vi "BodeFrequencyResponseAnalyzer.vi"() -> ()   [LabVIEW 2026]
doc: "Measures the magnitude and phase response of an electronic filter using synchronized analog generation and acquisition with NI-DAQmx."
uses:
  <vilib>/Utility/error.llb/DialogType.ctl
  <vilib>/DAQmx/create/channels.llb/DAQmx Create Channel (AI-Voltage-Basic).vi
  <vilib>/DAQmx/create/channels.llb/DAQmx Create Channel (AO-Voltage-Basic).vi
  <vilib>/DAQmx/configure/timing.llb/DAQmx Timing (Sample Clock).vi
  <vilib>/DAQmx/miscellaneous.llb/DAQmx Fill In Error Info.vi
  <vilib>/DAQmx/write.llb/DAQmx Write (Analog Wfm 1Chan NSamp).vi
  <vilib>/DAQmx/read.llb/DAQmx Read (Analog Wfm 1Chan NSamp).vi
  <vilib>/measure/NI_MABase.lvlib
  <resource>/objmgr/daqmx.rc
panel:
  out "Adaptive\nSamples\nTo Read":dbl
  in  "Minimum Cycles \nper Frequency":dbl=5.0 min=1.0 max=100.0 step=1.0
  in  "Sample Rate \n(samples/s)":dbl=40000.0 format="%#_13g"
  out "appended path":path
  in  "Select Saving Directory":path
  in  "Select Type Of Data":enum16{"BackLoopData.txt", "DUTData.txt"}(ring)
  out "Voltage Gain / Frequency":cluster{i32, dbl}[](graph)
  out "Amplitude":dbl
  out "Minimum\nSamples":dbl
  out "freq":i32
  in  "Max Frequency \nRange (1-10000 Hz)":i32=1000 min=1 max=10000 step=1
  out "Actual Sample Rate":dbl
  out "Chirp Signal (Output)":waveform(dbl)(graph)
  in  "Signal Type":T1(ring)
  in  "Amplitude (Volts)":dbl=1.0 format="%0.2p"
  in  "Input Channel":tag
  in  "stop":bool
  out "Filtered Signal (Input)":waveform(dbl)(graph)
  in  "Output  Channel":tag
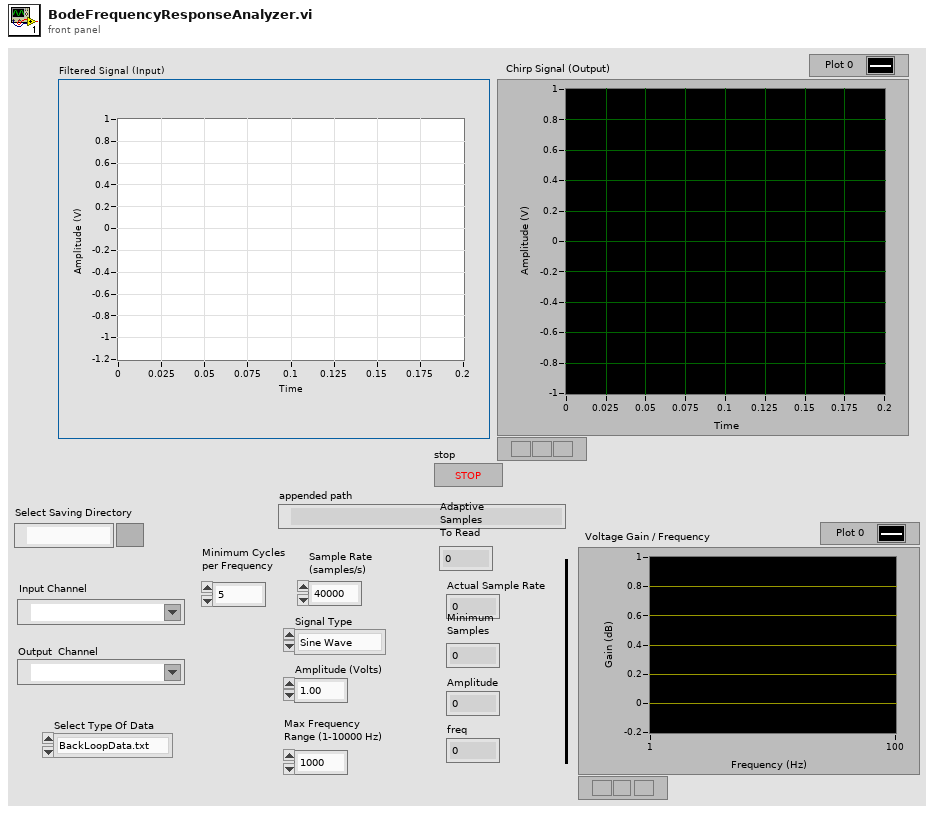
[diagram p1: front panel]
types:
  T1 = enum16{"Sine Wave", "Triangle Wave", "Square Wave", "Sawtooth Wave"}
  T2 = enum16{"open", "replace", "create", "open or create", "replace or create", "replace or create with confirmation"}
  T3 = typedef "DialogType.ctl" = u16
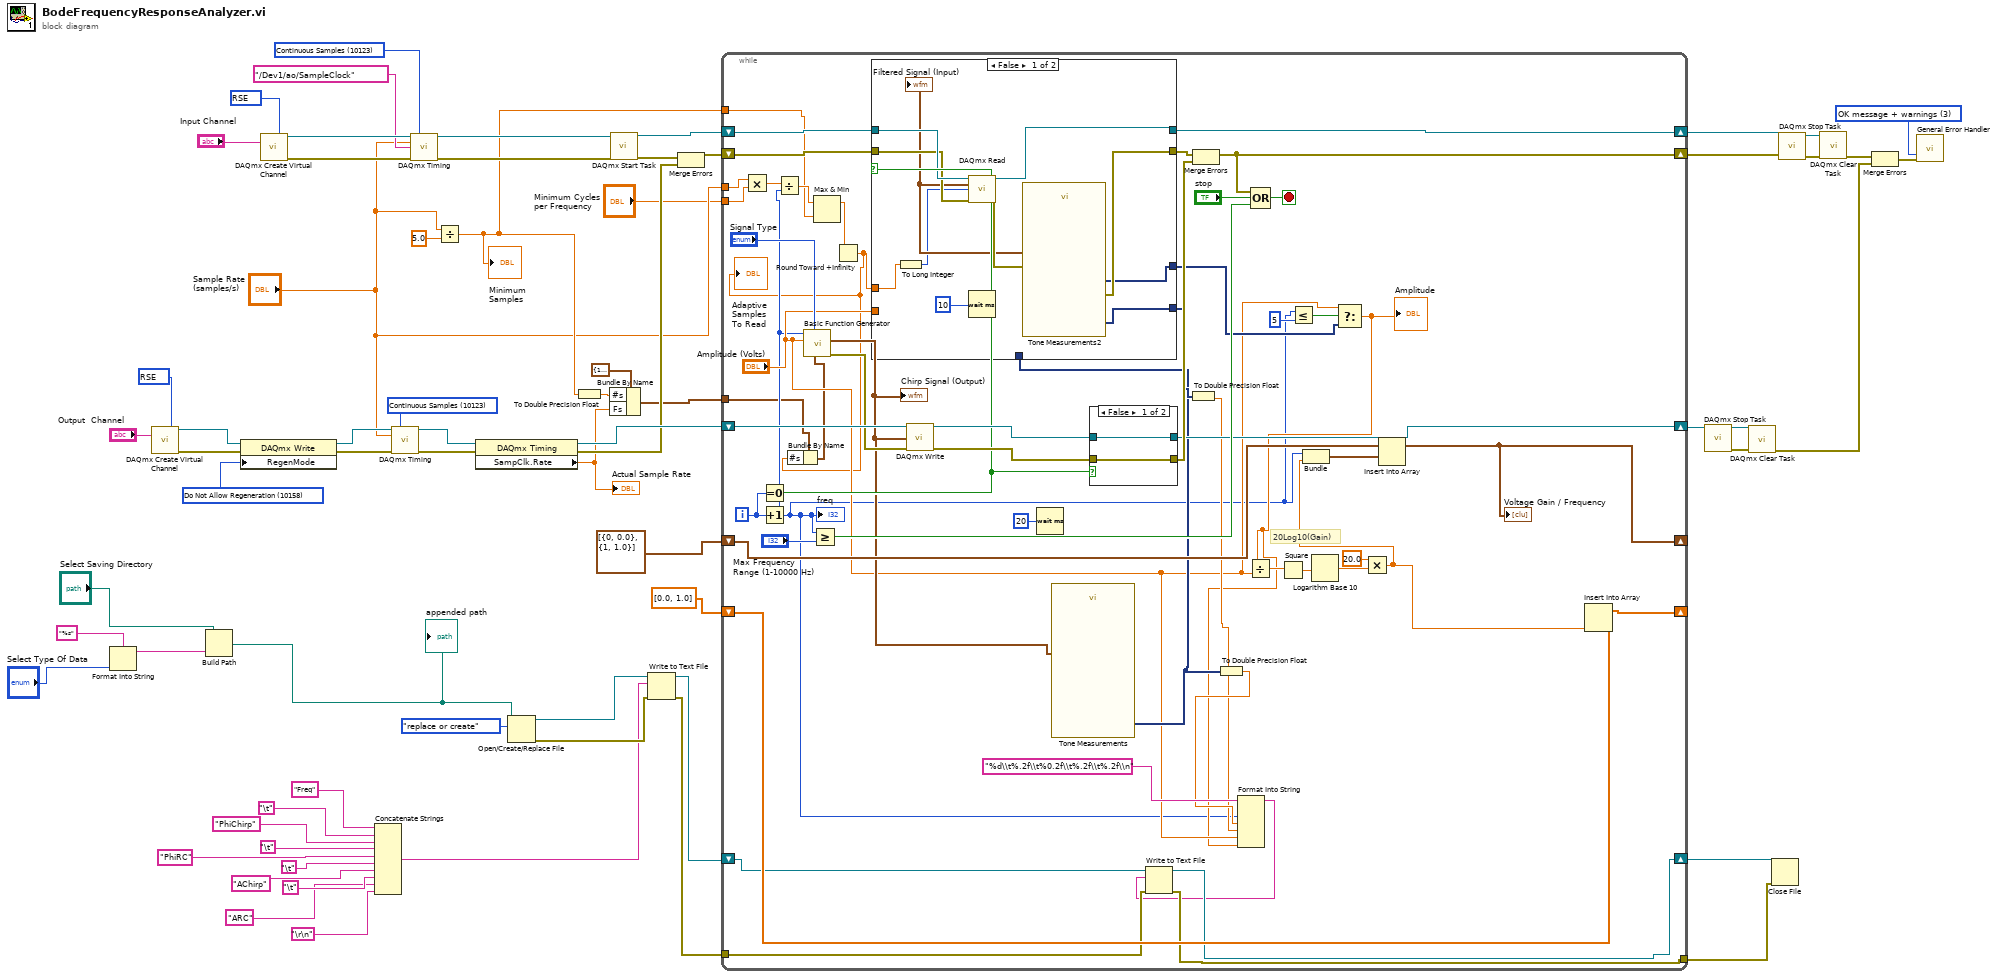
[diagram p0: block diagram]
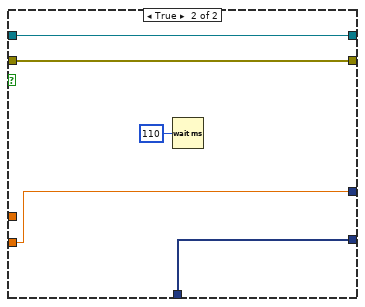
[diagram p2: hidden frame]
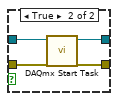
[diagram p3: hidden frame]
diagram:
  w28 = 10083 items=["Default"=-1, "RSE"=10083, "Differential"=10106, "Pseudodifferential"=12529] ("output terminal configuration")
  w29 = 10083 items=["Default"=-1, "RSE"=10083, "NRSE"=10078, "Differential"=10106, "Pseudodifferential"=12529] ("input terminal configuration")
  w45 = 10158 items=["Allow Regeneration"=10097, "Do Not Allow Regeneration"=10158] ("RegenMode")
  w51 = T3 3 items=["no dialog", "OK message", "continue or stop message", "OK message + warnings", "continue/stop + warnings"] ("type of dialog (OK msg:1)")
  w63 = 10123 items=["Finite Samples"=10178, "Continuous Samples"=10123, "Hardware Timed Single Point"=12522] ("sample mode")
  w66 = 10123 items=["Finite Samples"=10178, "Continuous Samples"=10123, "Hardware Timed Single Point"=12522] ("sample mode")
  n1 = Format Into String(format string="%s", "Select Type Of Data") -> (resulting string=w10:string)  [unwired: 2 in, 1 out]
  n2 = call-poly <vilib>:"DAQmx Create Virtual Channel.vi"("output terminal configuration"=w28, "physical channels"="Output  Channel") -> ("task out"=w49:refnum<k21>, "error out"=w48:errorcluster)  [unwired: 12 in]
  n3 = Build Path(base path="Select Saving Directory", name or relative path=w10) -> (appended path=w9:path)
  "appended path" <- w9
  n4 = property class="DAQmx Write"(reference=w49, error in=w48, "RegenMode"=w45) -> (reference out=w47:refnum<k21>, error out=w46:errorcluster)
  n5 = call-poly <vilib>:"DAQmx Create Virtual Channel.vi"("input terminal configuration"=w29, "physical channels"="Input Channel") -> ("task out"=w64:refnum<k21>, "error out"=w65:errorcluster)  [unwired: 12 in]
  n6 = Concatenate Strings("Freq" ("string"), "\t", "PhiChirp" ("string"), "\t", "PhiRC" ("string"), "\t", "AChirp" ("string"), "\t", "ARC" ("string"), "\r\n") -> (w14:string)
  n7 = call-poly <vilib>:"DAQmx Timing.vi"("task/channels in"=w47, "sample mode"=w66, "rate"="Sample Rate \n(samples/s)", "error in"=w46) -> ("task out"=w44:refnum<k21>, "error out"=w43:errorcluster)  [unwired: 10 in]
  n8 = call-poly <vilib>:"DAQmx Timing.vi"("task/channels in"=w64, "sample mode"=w63, "rate"="Sample Rate \n(samples/s)", "source"=tag "/Dev1/ao/SampleClock", "error in"=w65) -> ("task out"=w62:refnum<k21>, "error out"=w61:errorcluster)  [unwired: 9 in]
  n9 = Divide(x="Sample Rate \n(samples/s)", y=5.0) -> (x/y=w30:dbl)
  "Minimum\nSamples" <- w30
  n10 = property class="DAQmx Timing"(reference=w44, error in=w43) -> (reference out=w42:refnum<k21>, error out=w41:errorcluster, "SampClk.Rate"=w40:dbl)
  "Actual Sample Rate" <- w40
  n11 = Open/Create/Replace File(file path (use dialog)=w9, operation (0:open)=T2."replace or create") -> (refnum out=w22:refnum<file>, error out=w20:errorcluster)  [unwired: 4 in, 1 out]
  n12 = To Double Precision Float(number=w30) -> (double precision float=w38:dbl)
  n13 = Bundle By Name(cluster=cluster{"Fs":dbl, "#s":dbl} {"Fs"=1000.0, "#s"=1000.0} ("sampling info"), "#s"=w38, "Fs"=w40) -> (w37:cluster{"Fs":dbl, "#s":dbl})
  n14 = call <vilib>:"DAQmx Start Task.vi"("task/channels in"=w62, "error in"=w61) -> ("task out"=w59:refnum<k21>, "error out"=w34:errorcluster)  [unwired: 12 in]
  n15 = Write to Text File(file (use dialog)=w22, text=w14, error in=w20) -> (refnum out=w21:refnum<file>, error out=w19:errorcluster)  [unwired: 1 in, 1 out]
  n16 = Merge Errors(w34, w41) -> (w35:errorcluster)
  n17 = while {
    tunnel: w30 -> [w73]
    shift-right: [w99] -> w39
    shift-left: w42 -> [w119]
    shift-right: [w95] -> w33
    shift-left: w35 -> [w111]
    shift-right: [w121] -> w32
    shift-left: w59 -> [w122]
    tunnel: w37 -> [w71]
    shift-right: [w102] -> _
    shift-left: dbl[] [0.0, 1.0] -> [w97]
    shift-right: [w98] -> _
    shift-left: cluster{i32, dbl}[] [{0, 0.0}, {1, 1.0}] -> [w96]
    shift-right: [w87] -> w24
    shift-left: w21 -> [w88]
    tunnel: w19 -> [w84]
    tunnel: [w86] -> w23
    tunnel: "Sample Rate \n(samples/s)" -> [w69]
    tunnel: "Minimum Cycles \nper Frequency" -> [w77]
    i -> [w113]
    stop <- w116 stop-if-true
    # "20Log10(Gain)"
    n18 = Multiply(x=w69, y=w77) -> (x*y=w76:dbl)
    n19 = Equal To 0?(x=w113) -> (x = 0?=w112:bool)
    n20 = Increment(x=w113) -> (x+1=w75:i32)
    "freq" <- w75
    n21 = Divide(x=w76, y=w75) -> (x/y=w74:dbl)
    n22 = Greater Or Equal?(x=w75, y="Max Frequency \nRange (1-10000 Hz)") -> (x >= y?=w114:bool)
    n23 = Max & Min(x=w74, y=w73) -> (max(x,y)=w72:dbl)  [unwired: 1 out]
    n24 = Round Toward +Infinity(x=w72) -> (ceil(x): smallest int >= x=w68:dbl)
    "Adaptive\nSamples\nTo Read" <- w68
    n25 = Bundle By Name(cluster=w71, "#s"=w68) -> (w70:cluster{"Fs":dbl, "#s":dbl})
    n26 = call <vilib>:"Basic Function Generator.vi"("sampling info"=w70, "signal type"="Signal Type", "amplitude"="Amplitude (Volts)", "frequency"=w75) -> ("error out"=w110:errorcluster, "signal out"=w90:waveform(dbl))  [unwired: 5 in, 1 out]
    "Chirp Signal (Output)" <- w90
    n27 = call-poly <vilib>:"DAQmx Write.vi"("task/channels in"=w119, "data"=w90, "error in"=w110) -> ("task out"=w118:refnum<k21>, "error out"=w117:errorcluster)  [unwired: 10 in, 1 out]
    n28 = Wait (ms)(milliseconds to wait=u32 20) -> ()  [unwired: 1 out]
    n29 = call "Tone Measurements"("Signals"=w90) -> ("Phase"=w82:dynamicdata)  [unwired: 7 in, 3 out]
    n30 = case shown="False" w112 {
      tunnel: w122 -> [w133 w138]
      tunnel: [w132 w138] -> w121
      tunnel: [w129 w137] -> w109
      tunnel: w111 -> [w131 w137]
      tunnel: [w128 w136] -> w91
      tunnel: "Amplitude (Volts)" -> [_ w136]
      tunnel: [w125 w134] -> w89
      tunnel: w82 -> [_ w134]
      tunnel: w68 -> [w124 _]
      frame False {
        n31 = To Long Integer(number=w124) -> (32bit integer=w123:i32)
        n32 = call-poly <vilib>:"DAQmx Read.vi"("task/channels in"=w133, "number of samples per channel"=w123, "error in"=w131) -> ("task out"=w132:refnum<k21>, "data"=w126:waveform(dbl), "error out"=w130:errorcluster)  [unwired: 10 in]
        "Filtered Signal (Input)" <- w126
        n33 = Wait (ms)(milliseconds to wait=u32 10) -> ()  [unwired: 1 out]
        n34 = call "Tone Measurements2"("error in (no error)"=w130, "Signals"=w126) -> ("error out"=w129:errorcluster, "Phase"=w125:dynamicdata, "Amplitude"=w128:dynamicdata)  [unwired: 6 in, 1 out]
      }
      frame True {
        n35 = Wait (ms)(milliseconds to wait=u32 110) -> ()  [unwired: 1 out]
      }
    }
    n36 = case shown="False" w112 {
      tunnel: w118 -> [w140 w144]
      tunnel: w117 -> [w139 w143]
      tunnel: [w140 w142] -> w99
      tunnel: [w139 w141] -> w108
      frame False {
      }
      frame True {
        n37 = call <vilib>:"DAQmx Start Task.vi"("task/channels in"=w144, "error in"=w143) -> ("task out"=w142:refnum<k21>, "error out"=w141:errorcluster)  [unwired: 12 in]
      }
    }
    n38 = To Double Precision Float(number=w89) -> (double precision float=w80:dbl)
    n39 = Merge Errors(w109, w108) -> (w95:errorcluster)
    n40 = To Double Precision Float(number=w82) -> (double precision float=w81:dbl)
    n41 = Compound Arithmetic op=OR(w95, "stop", w114) -> (w116:bool)
    n42 = Less Or Equal?(x=w75, y=5) -> (x <= y?=w92:bool)
    n43 = Select(t="Amplitude (Volts)", s=w92, f=w91) -> (s? t:f=w78:dbl)
    "Amplitude" <- w78
    n44 = Format Into String(format string="%d\\t%.2f\\t%0.2f\\t%.2f\\t%.2f\\n", w75, w81, w80, "Amplitude (Volts)", w78) -> (resulting string=w83:string)  [unwired: 2 in, 1 out]
    n45 = Write to Text File(file (use dialog)=w88, text=w83, error in=w84) -> (refnum out=w87:refnum<file>, error out=w86:errorcluster)  [unwired: 1 in, 1 out]
    n46 = Divide(x=w78, y="Amplitude (Volts)") -> (x/y=w106:dbl)
    n47 = Square(x=w106) -> (x^2=w105:dbl)
    n48 = Logarithm Base 10(1:w105) -> (0:w104:dbl)
    n49 = Multiply(x=20.0, y=w104) -> (x*y=w101:dbl)
    n50 = Bundle(w75, w101) -> (w100:cluster{i32, dbl})  [unwired: 1 in]
    n51 = Insert Into Array(array=w96, new element=w100) -> (w98:cluster{i32, dbl}[])  [unwired: 1 in]
    "Voltage Gain / Frequency" <- w98
    n52 = Insert Into Array(array=w97, new element=w101) -> (w102:dbl[])  [unwired: 1 in]
  }
  n53 = call <vilib>:"DAQmx Stop Task.vi"("task/channels in"=w39) -> ("task out"=w57:refnum<k21>, "error out"=w56:errorcluster)  [unwired: 13 in]
  n54 = call <vilib>:"DAQmx Clear Task.vi"("task in"=w57, "error in"=w56) -> ("error out"=w55:errorcluster)  [unwired: 13 in]
  n55 = Close File(refnum=w24, error in=w23) -> ()  [unwired: 2 out]
  n56 = call <vilib>:"DAQmx Stop Task.vi"("task/channels in"=w32, "error in"=w33) -> ("task out"=w54:refnum<k21>, "error out"=w50:errorcluster)  [unwired: 12 in]
  n57 = call <vilib>:"DAQmx Clear Task.vi"("task in"=w54, "error in"=w50) -> ("error out"=w53:errorcluster)  [unwired: 13 in]
  n58 = Merge Errors(w53, w55) -> (w52:errorcluster)
  n59 = call <vilib>:"General Error Handler.vi"("type of dialog (OK msg:1)"=w51, "error in (no error)"=w52) -> ()  [unwired: 9 in, 5 out]
